vi "Draw_Cage_Outline_(round).vi"(3 "Error In":errorcluster, 5 "Bounding rectangle for cage outline, pix":T2, 6 "Picture refnum in":T1) -> (0 "Error Out":errorcluster, 2 "Picture refnum out":T1)   [LabVIEW 2018, in "Cage Diagram.lvlib"]
uses:
  Cage Diagram.lvlib
  <vilib>/vision/Image Controls.llb/IMAQ Image.ctl
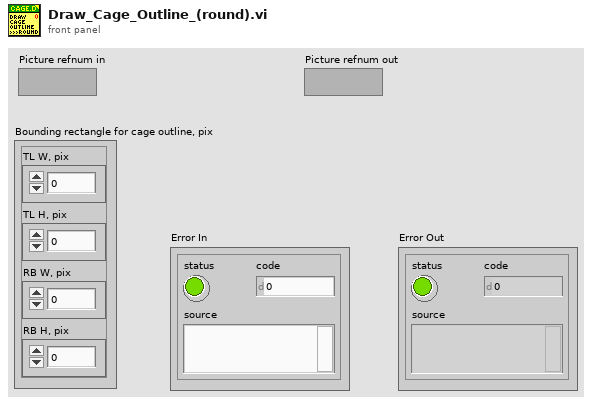
[diagram p1: front panel]
types:
  T1 = typedef "IMAQ Image.ctl" = refnum<image>
  T2 = cluster{"TL W, pix":i32, "TL H, pix":i32, "RB W, pix":i32, "RB H, pix":i32}
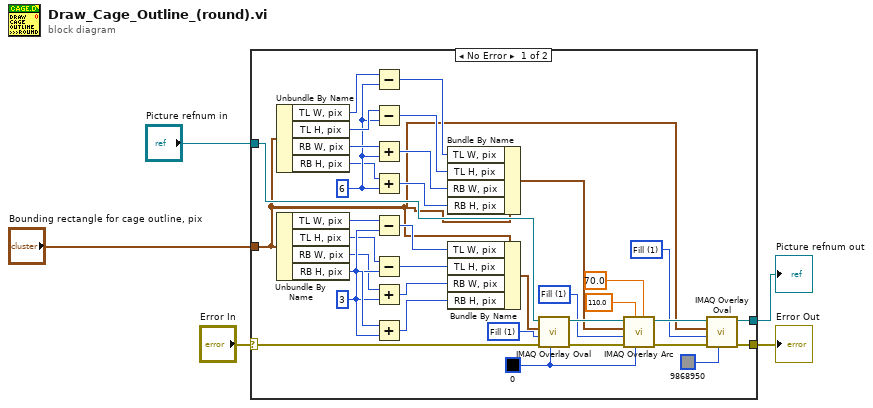
[diagram p0: block diagram]
diagram:
  n1 = case shown="No Error" "Error In" {
    selector: "Error In" -> [w15 w42]
    tunnel: [w10 w43] -> w4
    tunnel: "Picture refnum in" -> [w16 w43]
    tunnel: "Bounding rectangle for cage outline, pix" -> [w8 _]
    tunnel: [w11 w42] -> w1
    frame No Error {
      w9 = u32 1 items=["Frame", "Fill"] ("Drawing Mode (Frame)")
      w28 = u32 1 items=["Frame", "Fill"] ("Drawing Mode (Frame)")
      w35 = 6 ("y")
      w7 = u32 0 ("Color")
      w27 = u32 1 items=["Frame", "Fill"] ("Drawing Mode (Frame)")
      w20 = 3 ("y")
      n2 = Unbundle By Name(w8) -> ("TL W, pix"=w38:i32, "TL H, pix"=w37:i32, "RB W, pix"=w36:i32, "RB H, pix"=w34:i32)
      n3 = Unbundle By Name(w8) -> ("TL W, pix"=w17:i32, "TL H, pix"=w18:i32, "RB W, pix"=w19:i32, "RB H, pix"=w21:i32)
      n4 = Subtract(x=w38, y=w35) -> (x-y=w33:i32)
      n5 = Subtract(x=w37, y=w35) -> (x-y=w32:i32)
      n6 = Add(x=w36, y=w35) -> (x+y=w31:i32)
      n7 = Add(x=w34, y=w35) -> (x+y=w30:i32)
      n8 = Subtract(x=w17, y=w20) -> (x-y=w22:i32)
      n9 = Subtract(x=w18, y=w20) -> (x-y=w23:i32)
      n10 = Add(x=w19, y=w20) -> (x+y=w24:i32)
      n11 = Add(x=w21, y=w20) -> (x+y=w25:i32)
      n12 = Bundle By Name(cluster=w8, "TL W, pix"=w33, "TL H, pix"=w32, "RB W, pix"=w31, "RB H, pix"=w30) -> (w29:T2)
      n13 = Bundle By Name(cluster=w8, "TL W, pix"=w22, "TL H, pix"=w23, "RB W, pix"=w24, "RB H, pix"=w25) -> (w26:T2)
      n14 = call "IMAQ Overlay Oval"("Color"=w7, "error in (no error)"=w15, "Drawing Mode (Frame)"=w27, "Bounding Rectangle"=w26, "Image"=w16) -> ("error out"=w14:errorcluster, "Image Out"=w39:T1)  [unwired: 5 in]
      n15 = call "IMAQ Overlay Arc"("End Angle (degrees)"=70.0, "Color"=w7, "Start Angle (degrees)"=110.0, "error in (no error)"=w14, "Drawing Mode (Frame)"=w28, "Bounding Rectangle"=w29, "Image"=w39) -> ("error out"=w13:errorcluster, "Image Out"=w12:T1)  [unwired: 3 in]
      n16 = call "IMAQ Overlay Oval"("Color"=u32 9868950, "error in (no error)"=w13, "Drawing Mode (Frame)"=w9, "Bounding Rectangle"=w8, "Image"=w12) -> ("error out"=w11:errorcluster, "Image Out"=w10:T1)  [unwired: 5 in]
    }
    frame Error {
    }
  }
  "Error Out" <- w1
  "Picture refnum out" <- w4
